vi "Sub_VI-Sensores_Pressao.vi"(6 "Funcional/Estragado":bool, 7 "Densidade do líquido":dbl, 8 "Havia Furo Antes?":bool, 9 "Altura do sensor":i32, 10 "Altura Prevista":dbl, 11 "Altura Efetiva":dbl) -> (0 "Avariado":bool, 1 "Pressao":dbl, 2 "Furo no Tanque":bool, 3 "Sensor Ativado":bool)   [LabVIEW 2019]
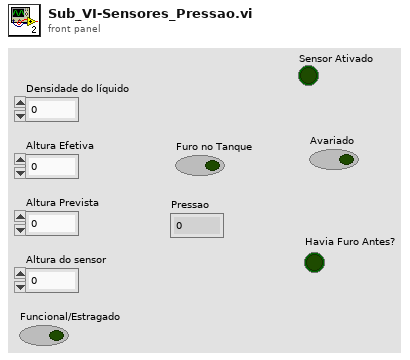
[diagram p1: front panel]
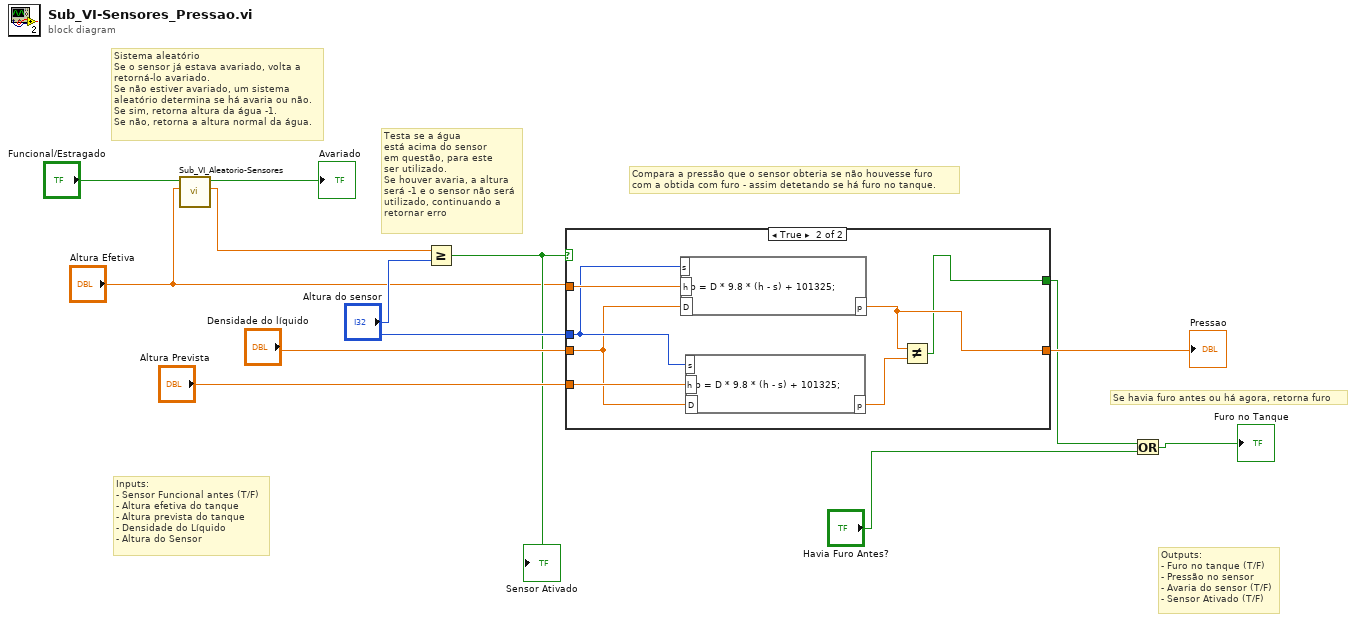
[diagram p0: block diagram]
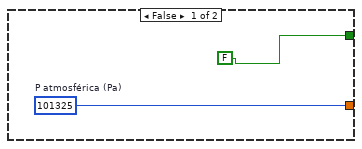
[diagram p2: hidden frame]
diagram:
  # "Se havia furo antes ou há agora, retorna furo"
  # "Inputs:\n- Sensor Funcional antes (T/F)\n- Altura efetiva do tanque\n- Altura prevista do tanque\n- Densidade do Líquido\n- Altura do Sensor"
  # "Outputs:\n- Furo no tanque (T/F)\n- Pressão no sensor\n- Avaria do sensor (T/F)\n- Sensor Ativado (T/F)"
  # "Compara a pressão que o sensor obteria se não houvesse furo\ncom a obtida com furo - assim detetando se há furo no tanque."
  # "Testa se a água\nestá acima do sensor\nem questão, para este\nser utilizado.\nSe houver avaria, a altura \nserá -1 e o sensor não será\nutilizado, continuando a \nretornar erro"
  # "Sistema aleatório\nSe o sensor já estava avariado, volta a\nretorná-lo avariado.\nSe não estiver avariado, um sistema \naleatório determina se há avaria ou não.\nSe sim, retorna altura da água -1.\nSe não, retorna a altura normal da água."
  n1 = call "Sub_VI_Aleatorio-Sensores.vi"("Altura da água"="Altura Efetiva", "Havia erro?"="Funcional/Estragado") -> ("Altura final água"=w7:dbl, "Boolean out"=→"Avariado":bool)  [unwired: 8 in]
  n2 = Greater Or Equal?(x=w7, y="Altura do sensor") -> (x >= y?=w5:bool)
  "Sensor Ativado" <- w5
  n3 = case shown="True" w5 {
    tunnel: "Altura Efetiva" -> [_ w19]
    tunnel: [w14 w20] -> w12
    tunnel: "Altura do sensor" -> [_ w17]
    tunnel: "Altura Prevista" -> [_ w18]
    tunnel: [FALSE w16] -> w3
    tunnel: "Densidade do líquido" -> [_ w15]
    frame False {
      w14 = 101325  # P atmosférica (Pa)
    }
    frame True {
      n4 = formula code="p = D * 9.8 * (h - s) + 101325;"("h"=w19, "s"=w17, "D"=w15) -> ("p"=w20:dbl)
      n5 = formula code="p = D * 9.8 * (h - s) + 101325;"("h"=w18, "s"=w17, "D"=w15) -> ("p"=w21:dbl)
      n6 = Not Equal?(x=w20, y=w21) -> (x != y?=w16:bool)
    }
  }
  "Pressao" <- w12
  n7 = Or(x=w3, y="Havia Furo Antes?") -> (x .or. y?=→"Furo no Tanque":bool)
